vi "GetAvailableFTDevices.vi"(8 "ErrorIn":errorcluster) -> (0 "ErrorOut":errorcluster, 1 "Descriptions":string[](array[string]), 2 "DevicesNr":i32, 3 "COMs":string[](array[string]))   [LabVIEW 2016]
doc: "Get all FTDI devices currently connected to the PC (array of serial port names, e.g. COM1) if there is such any one or throw error."
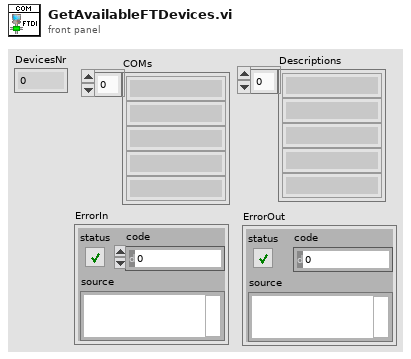
[diagram p1: front panel]
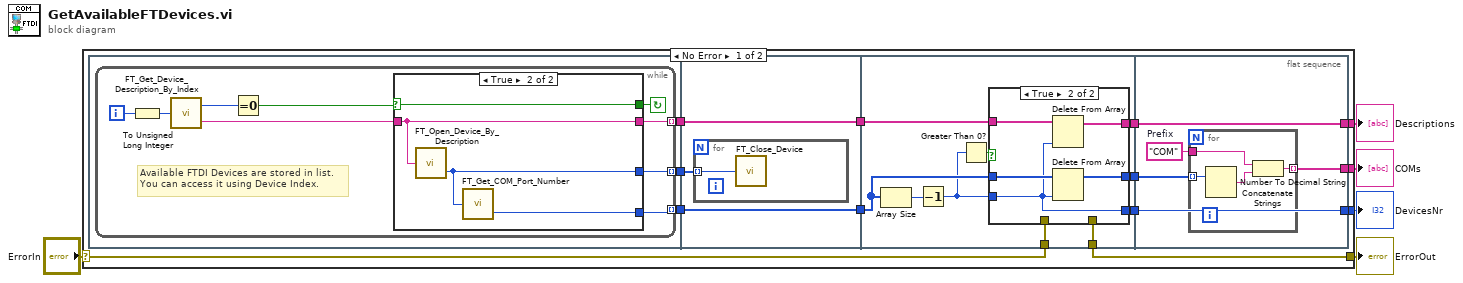
[diagram p0: block diagram]
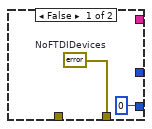
[diagram p3: hidden frame]
diagram:
  n1 = case shown="No Error" "ErrorIn" {
    selector: "ErrorIn" -> [w6 w66]
    tunnel: [w10 _] -> w5
    tunnel: [w9 _] -> w4
    tunnel: [w8 _] -> w3
    tunnel: [w7 w66] -> w2
    frame No Error {
      n2 = flat-sequence {
        tunnel: [w21] -> w18
        tunnel: [w20] -> w17
        tunnel: [w19] -> w16
        tunnel: w18 -> [w38]
        tunnel: w17 -> [w37]
        tunnel: w16 -> [w36]
        tunnel: [w37] -> w15
        tunnel: [w36] -> w14
        tunnel: w15 -> [w47]
        tunnel: w14 -> [w48]
        tunnel: [w49] -> w13
        tunnel: [w46] -> w12
        tunnel: [w43] -> w11
        tunnel: w6 -> [w42]
        tunnel: [w41] -> w7
        tunnel: [w60] -> w10
        tunnel: [w61] -> w8
        tunnel: w13 -> [w59]
        tunnel: w12 -> [w61]
        tunnel: w11 -> [w60]
        tunnel: [w57] -> w9
        frame #0 {
          n3 = while {
            tunnel: [w24] -> w21 mode=indexing
            tunnel: [w23] -> w20 mode=indexing
            tunnel: [w22] -> w19 mode=indexing
            i -> [w28]
            stop <- w25 continue-if-true
            # "Available FTDI Devices are stored in list.\nYou can access it using Device Index."
            n4 = To Unsigned Long Integer(number=w28) -> (unsigned 32bit integer=w26:u32)
            n5 = call "FT_Get_Device_Description_By_Index.vi"("Device Index"=w26) -> ("FT_Status"=w29:u32, "Device Description"=w27:string)
            n6 = Equal To 0?(x=w29) -> (x = 0?=w30:bool)
            n7 = case shown="True" w30 {
              selector: w30 -> [w31 w35]
              tunnel: w27 -> [_ w34]
              tunnel: [w31 w35] -> w25
              tunnel: [_ w34] -> w22
              tunnel: [_ w33] -> w24
              tunnel: [_ w32] -> w23
              frame False {
              }
              frame True {
                n8 = call "FT_Open_Device_By_Description.vi"("Device Description"=w34) -> ("Handle"=w33:u32)  [unwired: 1 out]
                n9 = call "FT_Get_COM_Port_Number.vi"("Handle"=w33) -> ("COM Port Number"=w32:i32)  [unwired: 1 out]
              }
            }
          }
        }
        frame #1 {
          n10 = for {
            tunnel: w38 -> [w39] mode=indexing
            n11 = call "FT_Close_Device.vi"("Handle"=w39) -> ()  [unwired: 1 out]
          }
        }
        frame #2 {
          n12 = Array Size(array=w47) -> (size(s)=w44:i32)
          n13 = Decrement(x=w44) -> (x-1=w40:i32)
          n14 = Greater Than 0?(x=w40) -> (x > 0?=w45:bool)
          n15 = case shown="True" w45 {
            tunnel: [_ w56] -> w49
            tunnel: w48 -> [_ w55]
            tunnel: w40 -> [_ w52]
            tunnel: w47 -> [_ w54]
            tunnel: [_ w53] -> w46
            tunnel: [0 w52] -> w43
            tunnel: w42 -> [_ _]
            tunnel: [w50 _] -> w41
            frame False {
              w50 = errorcluster {"status"=TRUE, "code"=-1, "source"="No available FTDI devices"}  # NoFTDIDevices
            }
            frame True {
              n16 = Delete From Array(array=w55, index=w52) -> (array with subset deleted=w53:string[])  [unwired: 1 in, 1 out]
              n17 = Delete From Array(array=w54, index=w52) -> (array with subset deleted=w56:i32[])  [unwired: 1 in, 1 out]
            }
          }
        }
        frame #3 {
          w58 = "COM"  # Prefix
          n18 = for {
            tunnel: w59 -> [w64] mode=indexing
            tunnel: w58 -> [w65]
            tunnel: [w62] -> w57 mode=indexing
            n19 = Number To Decimal String(number=w64) -> (decimal integer string=w63:string)  [unwired: 1 in]
            n20 = Concatenate Strings(w65, w63) -> (w62:string)
          }
        }
      }
    }
    frame Error {
    }
  }
  "DevicesNr" <- w5
  "COMs" <- w4
  "Descriptions" <- w3
  "ErrorOut" <- w2
